vi "Q14070-Z110下线，压铆调整螺塞.vi"() -> ()   [LabVIEW 2013]
uses:
  PCI8622_32.dll
panel:
  in  "确定按钮 3":bool
  in  "确定按钮 2":bool
  in  "密码":string
  in  "确定按钮":bool
  out "Y标尺最大值":dbl
  out "Y标尺最小值":dbl
  out "X标尺最大值":dbl
  out "X标尺最小值":dbl
  in  "员工权限":bool=TRUE
  out "error out 4":errorcluster
  out "型号数量":i32=10
  in  "产品ID":string
  in  "换向压力值":dbl=350.0 format="%#.2f"
  out "error out 3":errorcluster
  out "error out 2":errorcluster
  out "区域最大位移1(mm)":dbl format="%#.1f"
  out "区域最小位移1(mm)":dbl format="%#.1f"
  out "区域最大压力1(N)":dbl format="%#.3f"
  out "位移监控点1(mm)":dbl format="%#.1f"
  out "监控点最小压力1(N)":dbl format="%#.3f"
  out "监控点最大压力1(N)":dbl format="%#.3f"
  out "最小压入位移1(mm)":dbl format="%#.1f"
  out "最大压入位移1(mm)":dbl format="%#.1f"
  out "区域最小压力1(N)":dbl format="%#.3f"
  out "区域最小压力2(N)":dbl format="%#.3f"
  out "最小压入位移2(mm)":dbl format="%#.1f"
  out "最大压入位移2(mm)":dbl format="%#.1f"
  out "区域最大压力2(N)":dbl format="%#.3f"
  out "位移监控点2(mm)":dbl format="%#.1f"
  out "监控点最大压力2(N)":dbl format="%#.3f"
  out "监控点最小压力2(N)":dbl format="%#.3f"
  out "区域最小位移2(mm)":dbl format="%#.1f"
  out "区域最大位移2(mm)":dbl format="%#.1f"
  out "换向延时时间":dbl format="%#.1f"
  out "ADODB._Connection Out":refnum<k7>
  out "error out":errorcluster
  in  "联线按钮":bool
  out "通讯状态":bool
  in  "停止":bool
  in  "选项卡控件 2":enum32{"自动", "手动", "传感器校验", "参数查询"}(tab)
  out "上序不合格":bool
  out "上序合格":bool
  out "报警操作提示":string
  out "报警工步号":dbl
  out "扣铆":cluster{dbl[], dbl[]}[](graph)
  out "压装操作提示":string
  out "本工位合格":bool
  out "本工位不合格":bool
  in  "压装工步号":dbl
  out "位移(mm)":dbl format="%#.6f"
  out "压力(N)":dbl format="%#.4f"
  out "记号笔":bool
  out "急停":bool
  out "安全光幕":bool
  out "增压缸上位":bool
  out "顶升气缸下限":bool
  out "顶升气缸上限":bool
  in  "M顶转向器气缸下降":bool
  in  "M顶转向器气缸顶升":bool
  in  "M增压缸下降":bool
  in  "M增压缸上升":bool
  in  "M光幕屏蔽按钮":bool=TRUE
  in  "位移传感器零点偏移":dbl format="%#.2f"
  in  "位移传感器比例偏移":dbl=1.0 format="%#.2f"
  in  "压力传感器零点偏移":dbl=94.0 format="%#.2f"
  in  "压力传感器比例偏移":dbl=1.0 format="%#.2f"
  in  "传感器参数保存":bool
  in  "参数查询":bool
  in  "参数列表":string[][](table)
  in  "参数修改":bool
  out "员工ID":string
  out "员工姓名":string
  in  "型号选择":u16(ring)=1 items=["J706", "J709", "J728"]
  in  "参数加载":bool
  out "M延时暂存值":bool
  # "下线，压铆调整螺塞"
  # "Copying (C) 2015 湖北唯思凌科装备制造有限公司 版权所有"
  # "Q14070机械转向器装配线"
  # "传感器校验区"
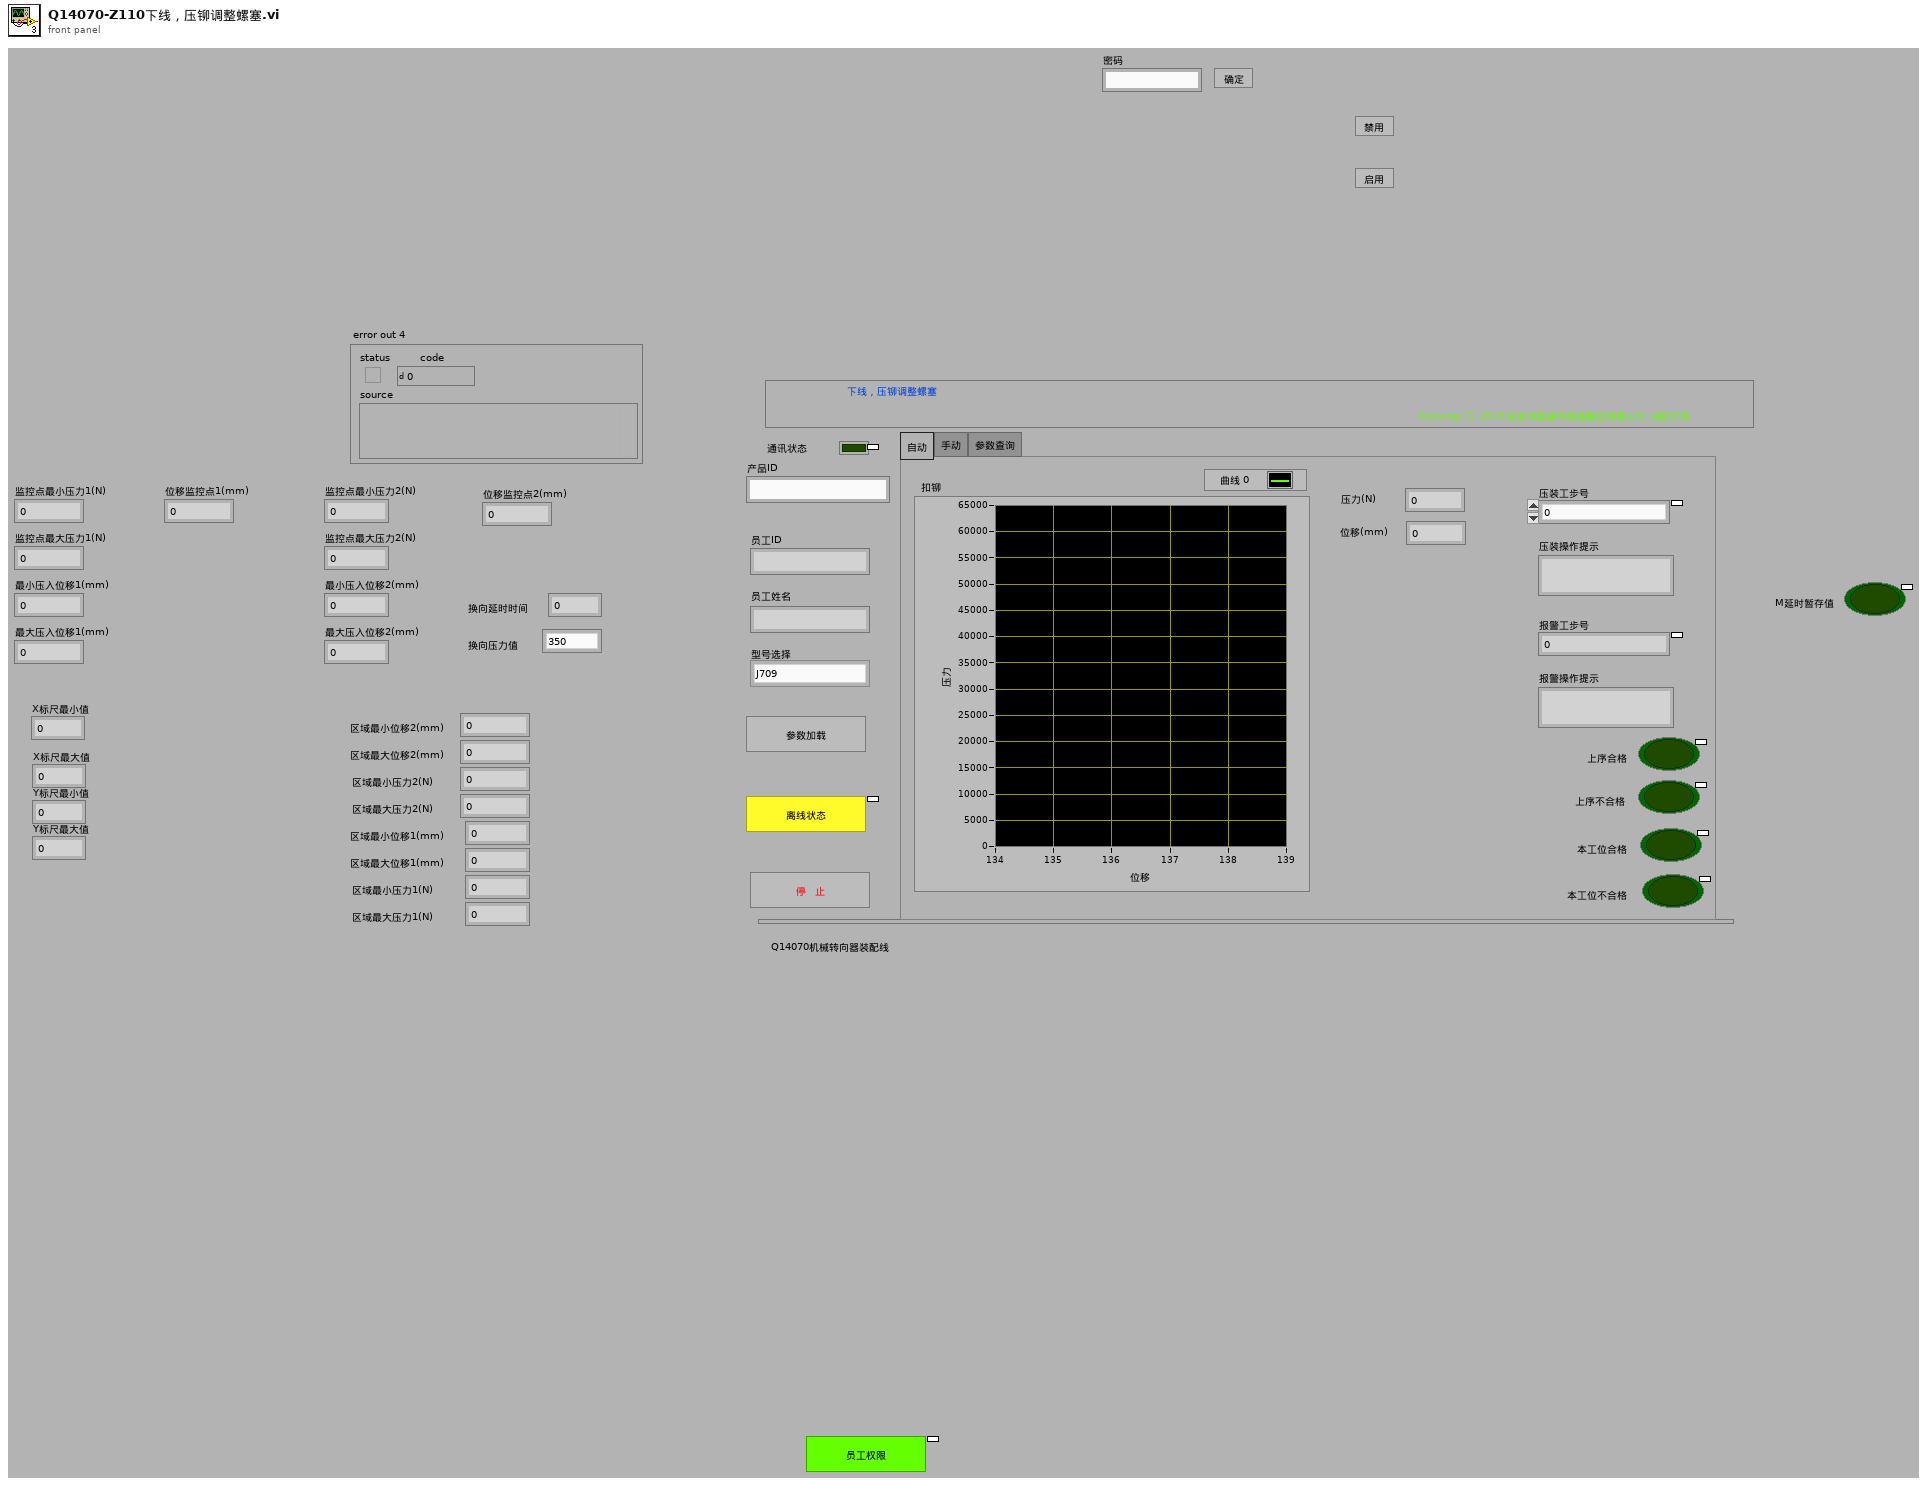
[diagram p1: front panel]
types:
  T1 = typedef "imagedata.ctl" = cluster{"image type":i32, "image depth":i32, "image":u8[], "mask":u8[], "colors":u32[], "Rectangle":cluster{"left":i16, "top":i16, "right":i16, "bottom":i16}}
  T2 = enum8{"Enabled", "Disabled", "Disabled and Grayed Out"}
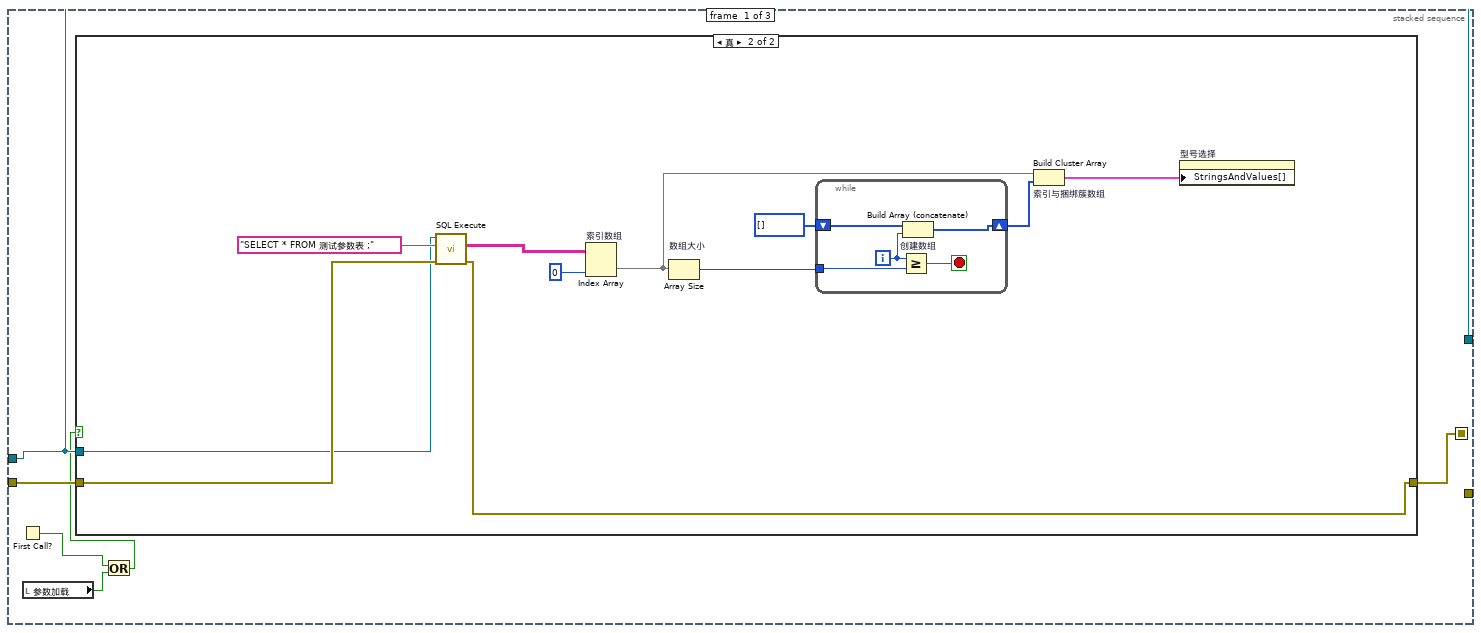
[diagram p3: hidden frame]
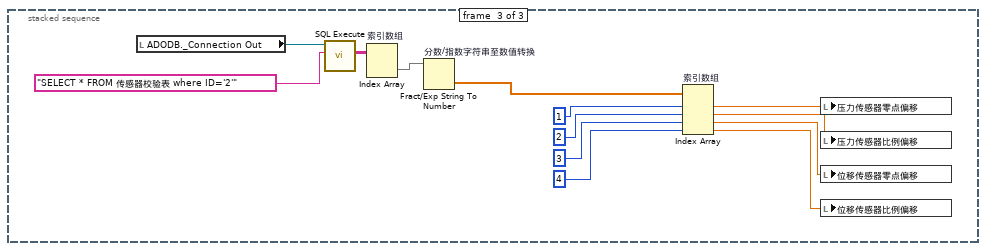
[diagram p5: hidden frame]
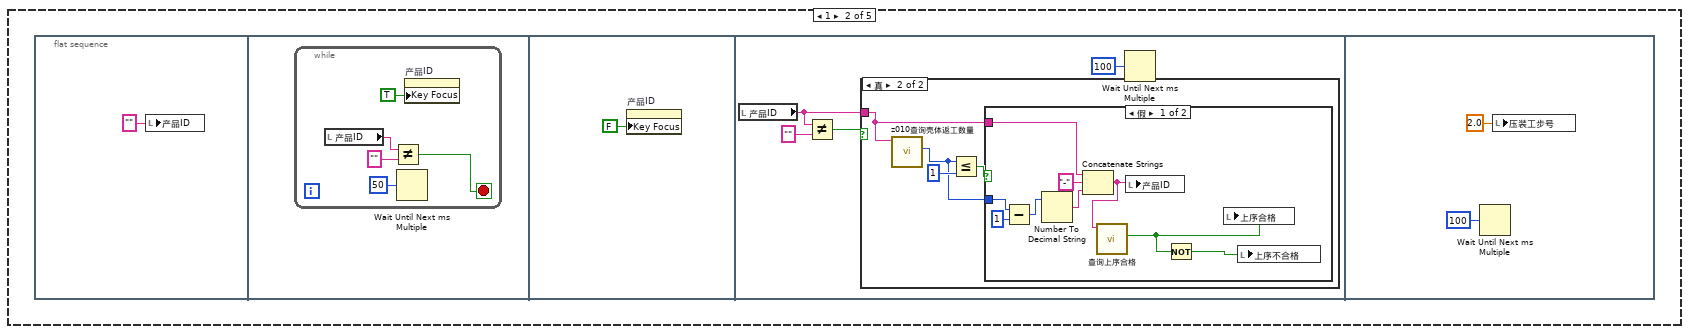
[diagram p7: hidden frame]
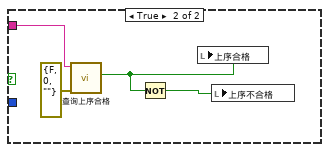
[diagram p9: hidden frame]
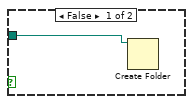
[diagram p12: hidden frame]
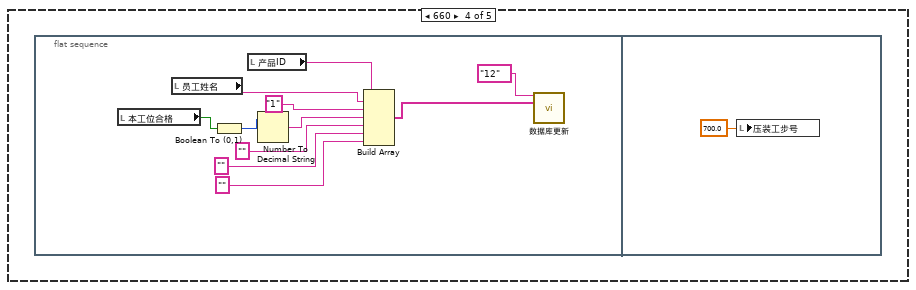
[diagram p13: hidden frame]
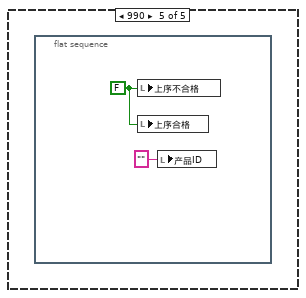
[diagram p14: hidden frame]
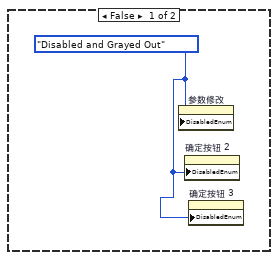
[diagram p15: hidden frame]
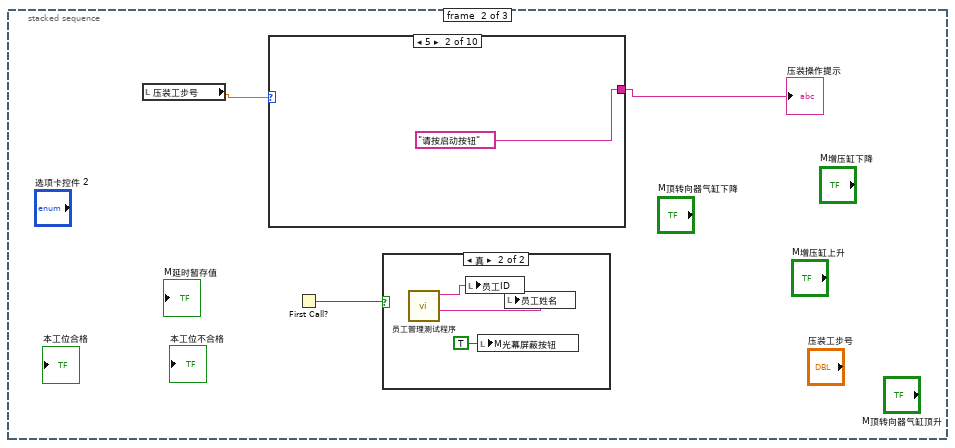
[diagram p20: hidden frame]
diagram:
  n1 = flat-sequence {
    tunnel: [w9] -> w4
    tunnel: [w8] -> w3
    tunnel: w4 -> [w16]
    tunnel: w3 -> [w15]
    tunnel: [w14] -> w2
    tunnel: [w13] -> w1
    tunnel: w2 -> [w131]
    tunnel: w1 -> [w130]
    frame #0 {
      n2 = call "ADO Connection Create.vi"() -> ("error out"=w11:errorcluster, "ADODB._Connection Out"=w12:refnum<k7>)  [unwired: 10 in]
      n3 = call "ADO Connection Open.vi"("error in (no error)"=w11, "ConnectionString"="DSN=参数Z110;", "ADODB._Connection In"=w12) -> ("error out"=w8:errorcluster, "ADODB._Connection Out"=w9:refnum<k7>)  [unwired: 7 in]
      "ADODB._Connection Out" <- w9
    }
    frame #1 {
      n4 = while {
        tunnel: w16 -> [w21]
        tunnel: w15 -> [w20]
        tunnel: [w19] -> w14
        tunnel: [w18] -> w13
        stop <- w24 stop-if-true
        n5 = local read "参数加载"() -> (w17:bool)
        n6 = Wait (ms)(milliseconds to wait=u32 100 ("等待时间（毫秒）")) -> ()  [unwired: 1 out]
        n7 = First Call?() -> (First Call?: T/F=w23:bool)
        n8 = Or(x=w23, y=w17) -> (x .or. y?=w22:bool)
        n9 = case shown="真" w22 {
          tunnel: w21 -> [w27 w31]
          tunnel: w20 -> [w26 w30]
          tunnel: [w27 w29] -> w19
          tunnel: [w26 w28] -> w18
          frame False {
          }
          frame True {
            n10 = stacked-sequence {
              seq-local: [w35 _ _] -> [_ w114 _]
              tunnel: w31 -> [w36 w111 _]
              tunnel: w30 -> [w37 _ _]
              tunnel: [w36 _ _] -> w29
              tunnel: [_ w113 _] -> w28
              frame #0 {
                n11 = First Call?() -> (First Call?: T/F=w34:bool)
                n12 = local read "参数加载"() -> (w33:bool)
                n13 = Or(x=w34, y=w33) -> (x .or. y?=w32:bool)
                n14 = case shown="真" w32 {
                  tunnel: w37 -> [w38 w43]
                  tunnel: w36 -> [_ w41]
                  tunnel: [w38 w40] -> w35
                  frame False {
                  }
                  frame True {
                    n15 = call "SQL Execute.vi"("error in (no error)"=w43, "Command Text"="SELECT * FROM 测试参数表 ;", "ADODB._Connection In"=w41) -> ("error out"=w40:errorcluster, "Data"=w44:string[][])  [unwired: 5 in, 2 out]
                    n16 = Index Array "索引数组"(array=w44, index (col)=0 ("禁用的索引 (列)")) -> (element=w47:string[])  [unwired: 1 in]
                    n17 = Array Size "数组大小"(array=w47) -> (size(s)=w46:i32)
                    n18 = while {
                      shift-right: [w52] -> w45
                      shift-left: i32[] [] -> [w53]
                      tunnel: w46 -> [w50]
                      i -> [w51]
                      stop <- w54 stop-if-true
                      n19 = Greater Or Equal?(x=w51, y=w50) -> (x >= y?=w54:bool)
                      n20 = Build Array (concatenate) "创建数组"(w53, w51) -> (w52:i32[])
                    }
                    n21 = Build Cluster Array "索引与捆绑簇数组"(w47, w45) -> (w39:cluster{"String":string, i32}[])
                    n22 = property on="型号选择" class="Ring (严格)"("StringsAndValues[]"=w39) -> ()  [unwired: 2 in, 2 out]
                  }
                }
              }
              frame #1 {
                n23 = property on="型号选择" class="Ring (严格)"() -> ("RingText.Text"=w110:string)  [unwired: 2 in, 2 out]
                n24 = call "创建文本2"("产品型号"=w110) -> ("Result"=w112:string)  [unwired: 13 in, 1 out]
                n25 = local write "M光幕屏蔽按钮"(TRUE ("M光幕屏蔽按钮")) -> ()
                n26 = call "SQL Execute.vi"("error in (no error)"=w114, "Command Text"=w112, "ADODB._Connection In"=w111) -> ("error out"=w113:errorcluster, "Data"=w116:string[][])  [unwired: 5 in, 2 out]
                n27 = Index Array "索引数组"(array=w116, index (row)=0 ("索引 (行)")) -> (element=w109:string[])  [unwired: 1 in]
                n28 = Fract/Exp String To Number "分数/指数字符串至数值转换"(string=w109) -> (number=w65:dbl[])  [unwired: 3 in, 1 out]
                n29 = local read "Y标尺最小值"() -> (w56:dbl)
                n30 = local read "X标尺最大值"() -> (w57:dbl)
                n31 = local read "X标尺最小值"() -> (w58:dbl)
                n32 = local read "Y标尺最大值"() -> (w55:dbl)
                n33 = property on="扣铆" class="XYGraph (严格)"("XScale.Minimum"=w58) -> ()  [unwired: 2 in, 2 out]
                n34 = property on="扣铆" class="XYGraph (严格)"("YScale.Minimum"=w56) -> ()  [unwired: 2 in, 2 out]
                n35 = property on="扣铆" class="XYGraph (严格)"("XScale.Maximum"=w57) -> ()  [unwired: 2 in, 2 out]
                n36 = property on="扣铆" class="XYGraph (严格)"("YScale.Maximum"=w55) -> ()  [unwired: 2 in, 2 out]
                n37 = Index Array(array=w65, index #1=1 ("索引"), index #2=2 ("索引"), index #3=3 ("索引"), index #4=4 ("索引"), index #5=5 ("索引"), index #6=6 ("索引"), index #7=7 ("索引"), index #8=8 ("索引"), index #9=9 ("索引"), index #10=10 ("索引"), index #11=11 ("索引"), index #12=12 ("索引"), index #13=13 ("索引"), index #14=14 ("索引"), index #15=15 ("索引"), index #16=16 ("索引"), index #17=17 ("索引"), index #18=18 ("索引"), index #19=19 ("索引"), index #20=20 ("索引"), index #21=21 ("索引"), index #22=22 ("索引"), index #23=23 ("索引"), index #24=24 ("索引")) -> (element #1=→"区域最小位移1(mm)":dbl, element #2=→"区域最大位移1(mm)":dbl, element #3=→"区域最小压力1(N)":dbl, element #4=→"区域最大压力1(N)":dbl, element #5=→"最小压入位移1(mm)":dbl, element #6=→"最大压入位移1(mm)":dbl, element #7=→"监控点最小压力1(N)":dbl, element #8=→"监控点最大压力1(N)":dbl, element #9=→"位移监控点1(mm)":dbl, element #10=→"区域最小位移2(mm)":dbl, element #11=→"区域最大位移2(mm)":dbl, element #12=→"区域最小压力2(N)":dbl, element #13=→"区域最大压力2(N)":dbl, element #14=→"最小压入位移2(mm)":dbl, element #15=→"最大压入位移2(mm)":dbl, element #16=→"监控点最小压力2(N)":dbl, element #17=→"监控点最大压力2(N)":dbl, element #18=→"位移监控点2(mm)":dbl, element #19=w64:dbl, element #20=→"换向延时时间":dbl, element #21=→"X标尺最小值":dbl, element #22=→"X标尺最大值":dbl, element #23=→"Y标尺最小值":dbl, element #24=→"Y标尺最大值":dbl)
                n38 = local write "换向压力值"(w64) -> ()
              }
              frame #2 {
                n39 = local read "ADODB._Connection Out"() -> (w124:refnum<k7>)
                n40 = call "SQL Execute.vi"("Command Text"="SELECT * FROM 传感器校验表 where ID='2'", "ADODB._Connection In"=w124) -> ("Data"=w129:string[][])  [unwired: 6 in, 3 out]
                n41 = Index Array "索引数组"(array=w129) -> (element=w128:string[])  [unwired: 2 in]
                n42 = Fract/Exp String To Number "分数/指数字符串至数值转换"(string=w128) -> (number=w127:dbl[])  [unwired: 3 in, 1 out]
                n43 = Index Array "索引数组"(array=w127, index #1=1 ("索引"), index #2=2 ("索引"), index #3=3 ("索引"), index #4=4 ("索引")) -> (element #1=w120:dbl, element #2=w119:dbl, element #3=w118:dbl, element #4=w117:dbl)
                n44 = local write "压力传感器零点偏移"(w120) -> ()
                n45 = local write "压力传感器比例偏移"(w119) -> ()
                n46 = local write "位移传感器零点偏移"(w118) -> ()
                n47 = local write "位移传感器比例偏移"(w117) -> ()
              }
            }
          }
        }
        n48 = local read "停止"() -> (w24:bool)
      }
    }
    frame #2 {
      n49 = call "ADO Connection Close.vi"("error in (no error)"=w130, "ADODB._Connection In"=w131) -> ("error out"=→"error out 2":errorcluster)  [unwired: 8 in, 1 out]
    }
  }
  n50 = while {
    stop <- w133 stop-if-true
    n51 = event shown="[2] \"参数修改\": 值改变" {
      selector: _ -> [_ _ _ _ _]
      dyn-events: _ -> [_ _ _ _ _]
      timeout: 500 -> [_ _ _ _ _]
      event Timeout {
        n52 = event-data() -> ()  [unwired: 3 out]
      }
      event "参数查询": Value Change {
        n53 = event-data() -> ()  [unwired: 7 out]
        n54 = flat-sequence {
          tunnel: [w144] -> w141
          tunnel: [w154] -> w140
          tunnel: [w150] -> w139
          tunnel: [w147] -> w138
          tunnel: w141 -> [w159]
          tunnel: w140 -> [w157]
          tunnel: [w158] -> w137
          tunnel: w139 -> [w158]
          tunnel: [w157] -> w136
          tunnel: w138 -> [w156]
          tunnel: w137 -> [w162]
          tunnel: w136 -> [w161]
          frame #0 {
            n55 = call "字符串转换为数组.vi"("查询内容"=",产品型号,区域最小位移1,区域最大位移1,区域最小压力1,区域最小压力1,最小压入位移1,最大压入位移1,监控点最小压力1,监控点最大压力1,位移监控点1,区域最小位移2,区域最大位移2,区域最小压力2,区域最小压力2,最小压入位移2,最大压入位移2,监控点最小压力2,监控点最大压力2,位移监控点2,换向压力,换向延时时间,X标尺最小值,X标尺最大值,Y标尺最小值,Y标尺最大值") -> ("列首"=w142:string[])  [unwired: 10 in]
            n56 = property on="参数列表" class="Tbl (严格)"("Row Headers[]"=w142) -> ()  [unwired: 2 in, 2 out]
          }
          frame #1 {
            n57 = call "创建文本"() -> ("Result"=w155:string)  [unwired: 14 in, 1 out]
            n58 = call "ADO Connection Create.vi"() -> ("error out"=w149:errorcluster, "ADODB._Connection Out"=w153:refnum<k7>)  [unwired: 10 in]
            n59 = call "ADO Connection Open.vi"("error in (no error)"=w149, "ConnectionString"="DSN=参数Z110;", "ADODB._Connection In"=w153) -> ("error out"=w148:errorcluster, "ADODB._Connection Out"=w151:refnum<k7>)  [unwired: 7 in]
            n60 = call "SQL Execute.vi"("error in (no error)"=w148, "Command Text"=w155, "ADODB._Connection In"=w151) -> ("error out"=w154:errorcluster, "Data"=w146:string[][], "ADODB._Connection Out"=w150:refnum<k7>)  [unwired: 5 in, 1 out]
            n61 = Transpose 2D Array "二维数组转置"(2D array=w146) -> (transposed array=w144:string[][])
            n62 = Index Array(array=w144, index (row)=0 ("索引 (行)")) -> (element=w147:string[])  [unwired: 1 in]
          }
          frame #2 {
            n63 = local write "参数列表"(w159) -> ()
            n64 = property on="参数列表" class="Tbl (严格)"("Column Headers[]"=w156) -> ()  [unwired: 2 in, 2 out]
          }
          frame #3 {
            n65 = call "ADO Connection Close.vi"("error in (no error)"=w161, "ADODB._Connection In"=w162) -> ("error out"=→"error out":errorcluster)  [unwired: 8 in, 1 out]
          }
        }
      }
      event "参数修改": Value Change {
        n66 = event-data() -> ()  [unwired: 7 out]
        n67 = while {
          i -> [w165]
          stop <- w172 stop-if-true
          n68 = local read "型号数量"() -> (w173:i32)
          n69 = local read "参数列表"() -> (w175:string[][])
          n70 = Greater Or Equal?(x=w165, y=w173) -> (x >= y?=w172:bool)
          n71 = Index Array(array=w175, index (col)=w165) -> (element=w174:string[])  [unwired: 1 in]
          n72 = stacked-sequence {
            seq-local: [w190 _] -> [_ w224]
            tunnel: w174 -> [w219 w233]
            tunnel: [_ w222] -> w163
            frame #0 {
              n73 = Index Array(array=w219, index #1=1 ("索引"), index #2=2 ("索引"), index #3=3 ("索引"), index #4=4 ("索引"), index #5=5 ("索引"), index #6=6 ("索引"), index #7=7 ("索引"), index #8=8 ("索引"), index #9=9 ("索引"), index #10=10 ("索引"), index #11=11 ("索引"), index #12=12 ("索引"), index #13=13 ("索引"), index #14=14 ("索引"), index #15=15 ("索引"), index #16=16 ("索引"), index #17=17 ("索引"), index #18=18 ("索引"), index #19=19 ("索引"), index #20=20 ("索引")) -> (element #1=w198:string, element #2=w197:string, element #3=w196:string, element #4=w195:string, element #5=w194:string, element #6=w193:string, element #7=w192:string, element #8=w191:string, element #9=w189:string, element #10=w188:string, element #11=w187:string, element #12=w186:string, element #13=w185:string, element #14=w184:string, element #15=w183:string, element #16=w182:string, element #17=w181:string, element #18=w180:string, element #19=w179:string, element #20=w178:string)
              n74 = call "创建文本6"("区域最小位移1"=w198, "区域最大位移1"=w197, "区域最小压力1"=w196, "区域最大压力1"=w195, "最小压入位移1"=w194, "最大压入位移1"=w193, "监控点最小压力1"=w192, "监控点最大压力1"=w191, "位移监控点1"=w189, "区域最小位移2"=w188, "区域最大位移2"=w187, "区域最小压力2"=w186, "区域最大压力2"=w185, "最小压入位移2"=w184, "最大压入位移2"=w183, "监控点最小压力2"=w182, "监控点最大压力2"=w181, "位移监控点2"=w180, "换向压力"=w179, "换向延时时间"=w178) -> ("Result"=w190:string)  [unwired: 6 in, 1 out]
            }
            frame #1 {
              n75 = Index Array(array=w233, index #1=21 ("索引"), index #2=22 ("索引"), index #3=23 ("索引"), index #4=24 ("索引"), index #5=0 ("索引")) -> (element #1=w221:string, element #2=w220:string, element #3=w227:string, element #4=w226:string, element #5=w225:string)
              n76 = call "创建文本5"("Y标尺最大值"=w226, "X标尺最小值"=w221, "X标尺最大值"=w220, "Y标尺最小值"=w227, "产品型号"=w225) -> ("Result"=w223:string)  [unwired: 9 in, 1 out]
              n77 = Concatenate Strings(w224, w223) -> (w222:string)
            }
          }
          n78 = call "ADO Connection Create.vi"("error in (no error)"=errorcluster {"status"=FALSE, "code"=0, "source"=""}) -> ("error out"=w169:errorcluster, "ADODB._Connection Out"=w171:refnum<k7>)  [unwired: 9 in]
          n79 = call "ADO Connection Open.vi"("error in (no error)"=w169, "ConnectionString"="DSN=参数Z110;", "ADODB._Connection In"=w171) -> ("error out"=w168:errorcluster, "ADODB._Connection Out"=w170:refnum<k7>)  [unwired: 7 in]
          n80 = call "SQL Execute.vi"("error in (no error)"=w168, "Command Text"=w163, "ADODB._Connection In"=w170) -> ("error out"=w176:errorcluster, "ADODB._Connection Out"=w177:refnum<k7>)  [unwired: 5 in, 2 out]
          n81 = call "ADO Connection Close.vi"("error in (no error)"=w176, "ADODB._Connection In"=w177) -> ("error out"=→"error out 4":errorcluster)  [unwired: 8 in, 1 out]
        }
      }
      event "传感器参数保存": Value Change {
        n82 = event-data() -> ()  [unwired: 7 out]
        n83 = local read "压力传感器零点偏移"() -> (w237:dbl)
        n84 = local read "压力传感器比例偏移"() -> (w236:dbl)
        n85 = local read "位移传感器零点偏移"() -> (w235:dbl)
        n86 = local read "位移传感器比例偏移"() -> (w234:dbl)
        n87 = call "ADO Connection Create.vi"() -> ("error out"=w250:errorcluster, "ADODB._Connection Out"=w252:refnum<k7>)  [unwired: 10 in]
        n88 = Number To Fractional String(number=w237, precision (6)=i16 3 ("精度(6)")) -> (F-format string=w243:string)  [unwired: 2 in]
        n89 = Number To Fractional String(number=w236, precision (6)=i16 2 ("精度(6)")) -> (F-format string=w242:string)  [unwired: 2 in]
        n90 = Number To Fractional String(number=w235, precision (6)=i16 1 ("精度(6)")) -> (F-format string=w241:string)  [unwired: 2 in]
        n91 = Number To Fractional String(number=w234, precision (6)=i16 2 ("精度(6)")) -> (F-format string=w240:string)  [unwired: 2 in]
        n92 = call "创建文本3"("位移1比例偏移值"=w240, "压力1零点偏移值"=w243, "压力1比例偏移值"=w242, "位移1零点偏移值"=w241) -> ("Result"=w239:string)  [unwired: 10 in, 1 out]
        n93 = call "ADO Connection Open.vi"("error in (no error)"=w250, "ConnectionString"="DSN=参数Z110;", "ADODB._Connection In"=w252) -> ("error out"=w249:errorcluster, "ADODB._Connection Out"=w251:refnum<k7>)  [unwired: 7 in]
        n94 = call "SQL Execute.vi"("error in (no error)"=w249, "Command Text"=w239, "ADODB._Connection In"=w251) -> ("error out"=w253:errorcluster, "ADODB._Connection Out"=w254:refnum<k7>)  [unwired: 5 in, 2 out]
        n95 = call "ADO Connection Close.vi"("error in (no error)"=w253, "ADODB._Connection In"=w254) -> ("error out"=→"error out 3":errorcluster)  [unwired: 8 in, 1 out]
      }
      event "停止": Value Change {
        n96 = event-data() -> ()  [unwired: 7 out]
        n97 = flat-sequence {
          frame #0 {
            n98 = local write "压装工步号"(0.0 ("工步号")) -> ()
          }
          frame #1 {
            n99 = Wait Until Next ms Multiple(millisecond multiple=u32 1000 ("毫秒倍数")) -> ()  [unwired: 1 out]
          }
          frame #2 {
            n100 = Quit LabVIEW(quit? (T)=TRUE ("停止？(T)")) -> ()
          }
        }
      }
    }
    n101 = Wait Until Next ms Multiple(millisecond multiple=u32 50 ("毫秒倍数")) -> ()  [unwired: 1 out]
    n102 = local read "停止"() -> (w133:bool)
  }
  n103 = while {
    stop <- w260 stop-if-true
    n104 = local read "压装工步号"() -> (w258:dbl)
    n105 = case shown="10" w258 {
      frame 0, Default {
      }
      frame 1 {
        n106 = flat-sequence {
          frame #0 {
            n107 = local write "产品ID"("" ("产品ID")) -> ()
          }
          frame #1 {
            n108 = while {
              stop <- w263 stop-if-true
              n109 = local read "产品ID"() -> (w265:string)
              n110 = Not Equal?(x=w265, y="") -> (x != y?=w263:bool)
              n111 = Wait Until Next ms Multiple(millisecond multiple=u32 50 ("毫秒倍数")) -> ()  [unwired: 1 out]
              n112 = property on="产品ID" class="Str"("Key Focus"=TRUE ("键选中")) -> ()  [unwired: 2 in, 2 out]
            }
          }
          frame #2 {
            n113 = property on="产品ID" class="Str"("Key Focus"=FALSE ("键选中")) -> ()  [unwired: 2 in, 2 out]
          }
          frame #3 {
            n114 = local read "产品ID"() -> (w269:string)
            n115 = Not Equal?(x=w269, y="") -> (x != y?=w270:bool)
            n116 = case shown="真" w270 {
              tunnel: w269 -> [_ w273]
              frame False {
              }
              frame True {
                n117 = call "z010查询壳体返工数量.vi"("转向器总成ID"=w273) -> ("Rows Fetched"=w272:i32)  [unwired: 8 in, 2 out]
                n118 = Less Or Equal?(x=w272, y=1) -> (x <= y?=w274:bool)
                n119 = case shown="假" w274 {
                  tunnel: w273 -> [w279 w285]
                  tunnel: w272 -> [w283 _]
                  frame False {
                    n120 = Subtract(x=w283, y=1) -> (x-y=w281:i32)
                    n121 = Number To Decimal String(number=w281) -> (decimal integer string=w284:string)  [unwired: 1 in]
                    n122 = Concatenate Strings(w279, "-" ("字符串"), w284) -> (w276:string)
                    n123 = call "查询上序合格.vi"("产品ID"=w276) -> ("上序合格"=w278:bool)  [unwired: 8 in, 2 out]
                    n124 = local write "产品ID"(w276) -> ()
                    n125 = Not(x=w278) -> (.not. x?=w277:bool)
                    n126 = local write "上序合格"(w278) -> ()
                    n127 = local write "上序不合格"(w277) -> ()
                  }
                  frame True {
                    n128 = call "查询上序合格.vi"("error in (no error)"=errorcluster {"status"=FALSE, "code"=0, "source"=""}, "产品ID"=w285) -> ("上序合格"=w288:bool)  [unwired: 7 in, 2 out]
                    n129 = Not(x=w288) -> (.not. x?=w286:bool)
                    n130 = local write "上序合格"(w288) -> ()
                    n131 = local write "上序不合格"(w286) -> ()
                  }
                }
              }
            }
            n132 = Wait Until Next ms Multiple(millisecond multiple=u32 100 ("毫秒倍数")) -> ()  [unwired: 1 out]
          }
          frame #4 {
            n133 = Wait Until Next ms Multiple(millisecond multiple=u32 100 ("毫秒倍数")) -> ()  [unwired: 1 out]
            n134 = local write "压装工步号"(2.0 ("压装工步号")) -> ()
          }
        }
      }
      frame 10 {
        n135 = flat-sequence {
          tunnel: [w297] -> w294
          tunnel: [w296] -> w293
          tunnel: w294 -> [w329]
          tunnel: w293 -> [w328]
          tunnel: [w329] -> w292
          tunnel: [w328] -> w291
          tunnel: w292 -> [w361]
          tunnel: w291 -> [w360]
          frame #0 {
            w295 = FALSE ("压装合格")
            n136 = local write "本工位不合格"(w295) -> ()
            n137 = local write "M延时暂存值"(w295) -> ()
            n138 = local write "本工位合格"(w295) -> ()
          }
          frame #1 {
            w298 = dbl[] [] ("添加的数组")
            n139 = while {
              shift-right: [w315] -> w297
              shift-left: w298 -> [w317]
              shift-right: [w314] -> w296
              shift-left: w298 -> [w316]
              stop <- w299 stop-if-true
              (unwired) "区域2"
              (unwired) "区域1"
              n140 = local read "区域最大位移2(mm)"() -> (w304:dbl)
              n141 = local read "区域最小位移2(mm)"() -> (w305:dbl)
              n142 = local read "区域最大压力2(N)"() -> (w302:dbl)
              n143 = local read "区域最小压力2(N)"() -> (w303:dbl)
              n144 = local read "区域最小位移1(mm)"() -> (w309:dbl)
              n145 = local read "区域最大位移1(mm)"() -> (w308:dbl)
              n146 = local read "区域最大压力1(N)"() -> (w306:dbl)
              n147 = local read "区域最小压力1(N)"() -> (w307:dbl)
              n148 = local read "位移(mm)"() -> (w321:dbl)
              n149 = local read "压力(N)"() -> (w318:dbl)
              n150 = Multiply(x=w321, y=1.0) -> (x*y=w319:dbl)
              n151 = call "区域曲线.vi"("区域最大压力(N)"=w302, "区域最小压力(N)"=w303, "区域最大位移(mm)"=w304, "区域最小位移(mm)"=w305) -> ("区域曲线"=w310:cluster{dbl[], dbl[]})  [unwired: 7 in]
              n152 = call "区域曲线.vi"("区域最大压力(N)"=w306, "区域最小压力(N)"=w307, "区域最大位移(mm)"=w308, "区域最小位移(mm)"=w309) -> ("区域曲线"=w311:cluster{dbl[], dbl[]})  [unwired: 7 in]
              n153 = Build Array (concatenate)(w316, w318) -> (w314:dbl[])
              n154 = Build Array (concatenate)(w317, w319) -> (w315:dbl[])
              n155 = Bundle(w315, w314) -> (w300:cluster{dbl[], dbl[]})  [unwired: 1 in]
              n156 = Wait Until Next ms Multiple(millisecond multiple=u32 50 ("毫秒倍数")) -> ()  [unwired: 1 out]
              n157 = Build Array(w300, w311, w310) -> (→"扣铆":cluster{dbl[], dbl[]}[])
              n158 = disable-structure shown="禁用" {
                frame Disabled {
                  n159 = local read "换向压力值"() -> (w324:dbl)
                  n160 = local read "压力(N)"() -> (w325:dbl)
                  n161 = Greater Or Equal?(x=w325, y=w324) -> (x >= y?=w323:bool)
                  n162 = case shown="真" w323 {
                    frame False {
                    }
                    frame True {
                      n163 = flat-sequence {
                        frame #0 {
                          n164 = Wait (ms)(milliseconds to wait=u32 1000 ("毫秒倍数")) -> ()  [unwired: 1 out]
                        }
                        frame #1 {
                          n165 = local write "M延时暂存值"(TRUE ("M延时暂存值")) -> ()
                        }
                      }
                    }
                  }
                }
                frame Enabled {
                }
              }
              n166 = local read "压装工步号"() -> (w313:dbl)
              n167 = Greater Or Equal?(x=w313, y=30.0) -> (x >= y?=w299:bool)
            }
          }
          frame #2 {
            n168 = local read "区域最大位移2(mm)"() -> (w335:dbl)
            n169 = local read "区域最小位移2(mm)"() -> (w336:dbl)
            n170 = local read "区域最大压力2(N)"() -> (w333:dbl)
            n171 = local read "区域最小压力2(N)"() -> (w334:dbl)
            n172 = local read "区域最小位移1(mm)"() -> (w340:dbl)
            n173 = local read "区域最大位移1(mm)"() -> (w339:dbl)
            n174 = local read "区域最大压力1(N)"() -> (w337:dbl)
            n175 = local read "区域最小压力1(N)"() -> (w338:dbl)
            n176 = Wait (ms)(milliseconds to wait=u32 100 ("毫秒倍数")) -> ()  [unwired: 1 out]
            n177 = call "区域判断.vi"("压力数组"=w328, "位移数组"=w329, "区域最大压力"=w337, "区域最小压力"=w338, "区域最大位移"=w339, "区域最小位移"=w340) -> ("区域监控合格"=w332:bool)  [unwired: 3 in]
            n178 = call "区域判断.vi"("压力数组"=w328, "位移数组"=w329, "区域最大压力"=w333, "区域最小压力"=w334, "区域最大位移"=w335, "区域最小位移"=w336) -> ("区域监控合格"=w331:bool)  [unwired: 3 in]
            n179 = And(x=w332, y=w331) -> (x .and. y?=w330:bool)
            n180 = Not(x=w330) -> (.not. x?=w341:bool)
            n181 = local write "本工位不合格"(w341) -> ()
            n182 = local write "本工位合格"(w330) -> ()
          }
          frame #3 {
            (unwired) "数据上传"
            n183 = flat-sequence {
              tunnel: [w371] -> w357
              tunnel: [w368] -> w356
              tunnel: [w365] -> w355
              tunnel: [w363] -> w354
              tunnel: w357 -> [w379]
              tunnel: w356 -> [w378]
              tunnel: w355 -> [w377]
              tunnel: ["F:\\报表储存\\"] -> w353
              tunnel: [w379] -> w352
              tunnel: [w376] -> w351
              tunnel: [w378] -> w350
              tunnel: [w376] -> w349
              tunnel: [w377] -> w348
              tunnel: [w376] -> w347
              tunnel: [w375] -> w346
              tunnel: w354 -> [w375]
              tunnel: w353 -> [w394]
              tunnel: w352 -> [w393]
              tunnel: w351 -> [w392]
              tunnel: w350 -> [w391]
              tunnel: w349 -> [w390]
              tunnel: w348 -> [w389]
              tunnel: w347 -> [w388]
              tunnel: [w386] -> w345
              tunnel: w346 -> [w383]
              tunnel: [w385] -> w344
              tunnel: w345 -> [w396]
              tunnel: w344 -> [w395]
              tunnel: [w395] -> w343
              tunnel: w343 -> [w399]
              frame #0 {
                n184 = local read "产品ID"() -> (w364:string)
                n185 = Format Date/Time String(time format string (%c)="%Y%m%d") -> (date/time string=w362:string)  [unwired: 2 in]
                n186 = String Subset(string=w362, offset (0)=6 ("偏移量(0)"), length (rest)=2 ("长度（剩余）")) -> (substring=w365:string)
                n187 = String Subset(string=w362, offset (0)=0 ("偏移量(0)"), length (rest)=4 ("长度（剩余）")) -> (substring=w371:string)
                n188 = String Subset(string=w362, offset (0)=4 ("偏移量(0)"), length (rest)=2 ("长度（剩余）")) -> (substring=w368:string)
                n189 = call <vilib>:"Trim Whitespace.vi"("string"=w364) -> ("trimmed string"=w363:string)  [unwired: 1 in]
              }
              frame #1 {
                w376 = "\\"
              }
              frame #2 {
                n190 = Concatenate Strings(w394, w393, w392, w391, w390, w389, w388) -> (w387:string)
                n191 = Concatenate Strings(w394, w393, w392, w391, w390, w389, w388) -> (w384:string)
                n192 = String To Path(string=w387) -> (path=w386:path)
                n193 = Concatenate Strings(w384, w383, ".JPG") -> (w381:string)
                n194 = String To Path(string=w381) -> (path=w385:path)
              }
              frame #3 {
                n195 = call <vilib>:"Check if File or Folder Exists.vi"("path"=w396) -> ("file or folder exists?"=w397:bool)  [unwired: 8 in, 2 out]
                n196 = case shown="真" w397 {
                  tunnel: w396 -> [w398 _]
                  frame False {
                    n197 = Create Folder(path (use dialog)=w398) -> ()  [unwired: 2 in, 3 out]
                  }
                  frame True {
                  }
                }
              }
              frame #4 {
                n198 = control-ref of="本VI"() -> (w401:refnum<vi>)
                n199 = invoke class="VI" method="FP.Get Image"(reference=w401) -> ("image data"=w400:T1)  [unwired: 5 in, 5 out]
                n200 = call <vilib>:"Write JPEG File.vi"("image data"=w400, "path to JPEG file"=w399) -> ()  [unwired: 8 in, 2 out]
              }
            }
            n201 = Build Array(w361, w360) -> (w359:dbl[][])
            n202 = call "数据存储.vi"("字符串"="E:\\sjcc\\", "2D data"=w359) -> ()  [unwired: 10 in]
          }
          frame #4 {
          }
        }
      }
      frame 660 {
        n203 = flat-sequence {
          frame #0 {
            n204 = local read "本工位合格"() -> (w410:bool)
            n205 = local read "员工姓名"() -> (w403:string)
            n206 = Boolean To (0,1)(Boolean=w410) -> (0, 1=w409:i16)
            n207 = local read "产品ID"() -> (w402:string)
            n208 = Number To Decimal String(number=w409) -> (decimal integer string=w408:string)  [unwired: 1 in]
            n209 = Build Array(w402, w403, "1" ("元素"), w408, "" ("元素"), "" ("元素"), "" ("元素")) -> (w404:string[])
            n210 = call "数据库更新.vi"("设备号"="12", "数据"=w404) -> ()  [unwired: 13 in, 1 out]
          }
          frame #1 {
            n211 = local write "压装工步号"(700.0 ("压装工步号")) -> ()
          }
        }
      }
      frame 990 {
        n212 = flat-sequence {
          frame #0 {
            w415 = FALSE ("M上序不合格")
            n213 = local write "上序不合格"(w415) -> ()
            n214 = local write "上序合格"(w415) -> ()
            n215 = local write "产品ID"("" ("产品ID")) -> ()
          }
        }
      }
    }
    n216 = Wait Until Next ms Multiple(millisecond multiple=u32 50 ("毫秒倍数")) -> ()  [unwired: 1 out]
    n217 = local read "停止"() -> (w260:bool)
  }
  n218 = while {
    stop <- w416 stop-if-true
    n219 = stacked-sequence {
      frame #0 {
        n220 = Equal?(x="密码", y="jizhuan") -> (x = y?=w420:bool)
        n221 = Compound Arithmetic op=AND(w420, "确定按钮") -> (w418:bool)
        n222 = case shown="真" w418 {
          frame False {
            w423 = T2."Disabled and Grayed Out" ("禁用")
            n223 = property on="参数修改" class="Bool"("DisabledEnum"=w423) -> ()  [unwired: 2 in, 2 out]
            n224 = property on="确定按钮 2" class="Bool"("DisabledEnum"=w423) -> ()  [unwired: 2 in, 2 out]
            n225 = property on="确定按钮 3" class="Bool"("DisabledEnum"=w423) -> ()  [unwired: 2 in, 2 out]
          }
          frame True {
            w424 = T2."Enabled" ("禁用")
            n226 = property on="参数修改" class="Bool"("DisabledEnum"=w424) -> ()  [unwired: 2 in, 2 out]
            n227 = property on="确定按钮 2" class="Bool"("DisabledEnum"=w424) -> ()  [unwired: 2 in, 2 out]
            n228 = property on="确定按钮 3" class="Bool"("DisabledEnum"=w424) -> ()  [unwired: 2 in, 2 out]
            n229 = case shown="真" "确定按钮 2" {
              frame False {
              }
              frame True {
                n230 = property on="选项卡控件 2" class="TabCtl (严格)"() -> ("Pages"=w434:refnum<vi>[])  [unwired: 2 in, 2 out]
                n231 = for {
                  N: 4 -> [_]
                  tunnel: w434 -> [w435] mode=indexing
                  i -> [w436]
                  n232 = case shown="2" w436 {
                    tunnel: w435 -> [_ w438]
                    frame 0, Default {
                    }
                    frame 2 {
                      n233 = property class="Page"(reference=w438, "PageVis"=FALSE ("选项卡可见")) -> ()  [unwired: 1 in, 2 out]
                    }
                  }
                }
              }
            }
            n234 = case shown="真" "确定按钮 3" {
              frame False {
              }
              frame True {
                n235 = property on="选项卡控件 2" class="TabCtl (严格)"() -> ("Pages"=w428:refnum<vi>[])  [unwired: 2 in, 2 out]
                n236 = for {
                  N: 4 -> [_]
                  tunnel: w428 -> [w429] mode=indexing
                  i -> [w430]
                  n237 = case shown="2" w430 {
                    tunnel: w429 -> [_ w432]
                    frame 0, Default {
                    }
                    frame 2 {
                      n238 = property class="Page"(reference=w432, "PageVis"=TRUE ("选项卡可见")) -> ()  [unwired: 1 in, 2 out]
                    }
                  }
                }
              }
            }
          }
        }
      }
      frame #1 {
        n239 = local read "压装工步号"() -> (w441:dbl)
        n240 = case shown="5" w441 {
          tunnel: [w446 "请按启动按钮" "增压缸下降" ("工步操作状态") "压装增压缸增压" ("工步操作状态") "增压缸保持3S后退回" ("工步操作状态") "顶转向器上升" ("工步操作状态") "顶转向器下降" "取记号笔" ("工步操作状态") "记号笔放回" ("工步操作状态") "循环结束" ("工步操作状态")] -> w440
          frame 0, Default {
            n241 = local read "联线按钮"() -> (w445:bool)
            n242 = case shown="假" w445 {
              tunnel: ["等待工件" ("工步操作状态") "等待扫描条码" ("工步操作状态")] -> w446
              frame False {
              }
              frame True {
              }
            }
          }
          frame 5 {
          }
          frame 10 {
          }
          frame 20 {
          }
          frame 30 {
          }
          frame 40 {
          }
          frame 50 {
          }
          frame 710 {
          }
          frame 720 {
          }
          frame 990 {
          }
        }
        "压装操作提示" <- w440
        n243 = First Call?() -> (First Call?: T/F=w439:bool)
        n244 = case shown="真" w439 {
          frame False {
          }
          frame True {
            n245 = call "员工管理测试程序.vi"() -> ("员工姓名"=w443:string, "员工ID"=w442:string)  [unwired: 10 in]
            n246 = local write "员工ID"(w442) -> ()
            n247 = local write "M光幕屏蔽按钮"(TRUE ("M光幕屏蔽按钮")) -> ()
            n248 = local write "员工姓名"(w443) -> ()
          }
        }
      }
      frame #2 {
        n249 = local read "报警工步号"() -> (w459:dbl)
        n250 = case shown="1" w459 {
          tunnel: ["无报警" "急停按钮被按下"] -> w458
          frame 0, Default {
          }
          frame 1 {
          }
        }
        "报警操作提示" <- w458
      }
    }
    n251 = Wait Until Next ms Multiple(millisecond multiple=u32 50 ("毫秒倍数")) -> ()  [unwired: 1 out]
    n252 = local read "停止"() -> (w416:bool)
  }
  n253 = flat-sequence {
    tunnel: [w462] -> w7
    tunnel: w7 -> [w464]
    tunnel: [w463] -> w6
    tunnel: w6 -> [w504]
    tunnel: [w504] -> w5
    tunnel: w5 -> [w506]
    frame #0 {
      n254 = call "PCI8622配置.vi"() -> ("DeviceID"=w462:i32)  [unwired: 11 in]
    }
    frame #1 {
      n255 = while {
        tunnel: w464 -> [w491]
        tunnel: [w491] -> w463
        stop <- "停止" stop-if-true
        w501 = 0  # nRetSizeWords
        w502 = 2048  # nReadSizeWords
        # "hDevice"
        n256 = Initialize Array(u16 0, 2048 ("dimension size")) -> (w492:u16[])
        n257 = dll-call lib="PCI8622_32.dll" fn="PCI8622_ReadDeviceProAD_Npt" label="ReadDeviceProAD_Npt"("hDevice"=w491, "ADBuffer[]"=w492, "nReadSizeWords"=w502, "nRetSizeWords"=w501) -> ("ADBuffer[]"=w495:u16[])  [unwired: 7 in, 2 out]
        n258 = Divide(x=w495, y=65536.01) -> (x/y=w496:dbl[])
        n259 = Multiply(x=w496, y=20) -> (x*y=w499:dbl[])
        n260 = Subtract(x=w499, y=10) -> (x-y=w485:dbl[])
        n261 = Decimate 1D Array "抽取一维数组"(w485) -> (w479:dbl[], w480:dbl[])  [unwired: 6 out]
        n262 = Add Array Elements(numeric array=w479) -> (sum=w486:dbl)
        n263 = Add Array Elements(numeric array=w480) -> (sum=w489:dbl)
        n264 = Array Size(array=w479) -> (size(s)=w487:i32)
        n265 = Array Size(array=w480) -> (size(s)=w488:i32)
        n266 = Divide(x=w486, y=w487) -> (x/y=w482:dbl)
        n267 = Divide(x=w489, y=w488) -> (x/y=w483:dbl)
        n268 = local read "位移传感器零点偏移"() -> (w468:dbl)
        n269 = local read "位移传感器比例偏移"() -> (w467:dbl)
        n270 = Multiply(x=25.0 ("y"), y=w483) -> (x*y=w469:dbl)
        n271 = Subtract(x=w482, y=0.0) -> (x-y=w478:dbl)
        n272 = local read "压力传感器零点偏移"() -> (w473:dbl)
        n273 = local read "压力传感器比例偏移"() -> (w471:dbl)
        n274 = Multiply(x=w478, y=10000.0) -> (x*y=w476:dbl)
        n275 = Subtract(x=w469, y=w468) -> (x-y=w466:dbl)
        n276 = Multiply(x=w466, y=w467) -> (x*y=→"位移(mm)":dbl)
        n277 = Add(x=w476, y=1.0) -> (x+y=w474:dbl)
        n278 = Subtract(x=w474, y=w473) -> (x-y=w472:dbl)
        n279 = Multiply(x=w472, y=w471) -> (x*y=→"压力(N)":dbl)
        n280 = Wait Until Next ms Multiple(millisecond multiple=u32 50 ("毫秒倍数")) -> ()  [unwired: 1 out]
      }
    }
    frame #2 {
      n281 = dll-call lib="PCI8622_32.dll" fn="PCI8622_StopDeviceProAD" label="StopDeviceProAD"("hDevice"=w504) -> ("hDevice"=w505:i32)  [unwired: 4 in, 2 out]
      n282 = dll-call lib="PCI8622_32.dll" fn="PCI8622_ReleaseDeviceProAD" label="ReleaseDeviceProAD"("hDevice"=w505) -> ()  [unwired: 5 in, 2 out]
    }
    frame #3 {
      n283 = dll-call lib="PCI8622_32.dll" fn="PCI8622_ReleaseDevice" label="ReleaseDevice"("hDevice"=w506) -> ()  [unwired: 5 in, 2 out]
    }
  }
